vi "MAVLink RC CH IN.vi"(7 "FGV Method":T2, 11 "RC CH IN":T1) -> (3 "RC CH IN out":T1)   [LabVIEW 2014]
uses:
  Controls/FGV Methods.ctl
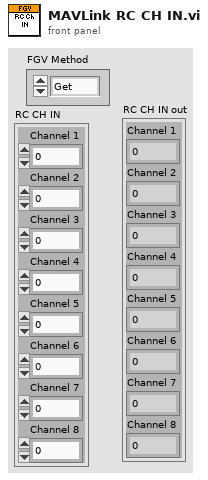
[diagram p1: front panel]
types:
  T1 = cluster{"Channel 1":u16, "Channel 2":u16, "Channel 3":u16, "Channel 4":u16, "Channel 5":u16, "Channel 6":u16, "Channel 7":u16, "Channel 8":u16}
  T2 = typedef "FGV Methods.ctl" = enum16{"Get", "Set"}
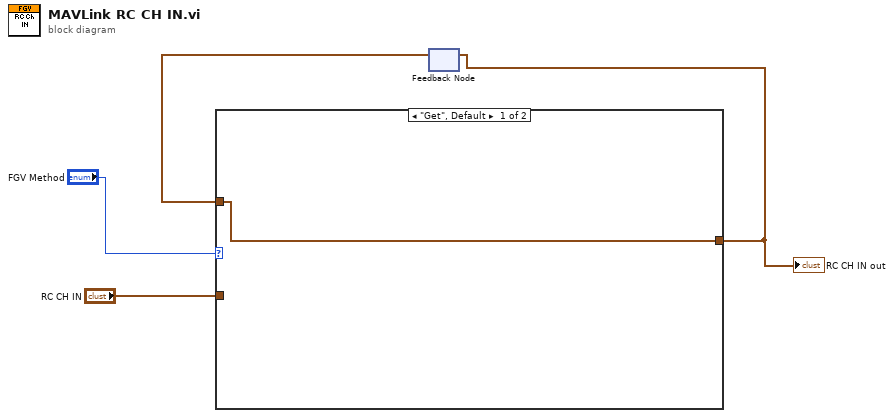
[diagram p0: block diagram]
diagram:
  n1 = feedback #1() -> (w2:T1)  [unwired: 1 in]
  n2 = case shown="\"Get\", Default" "FGV Method" {
    tunnel: "RC CH IN" -> [_ w6]
    tunnel: [w5 w6] -> w3
    tunnel: w2 -> [w5 _]
    frame "Get", Default {
    }
    frame "Set" {
    }
  }
  "RC CH IN out" <- w3
  n3 = feedback-in #1(w3) -> ()
